vi "deinitialize.vi"(0 "HGF_ImaqFg":refnum<class "HGF_ImaqFg.lvclass">, 5 "error in (no error)":errorcluster) -> (19 "error out":errorcluster)   [LabVIEW 2014, in "HGF_IMAQ.lvlib" / "HGF_ImaqFg.lvclass"]
doc: "This is a dynamic dispatch VI. It can be overwritten by childclasses to release allocated recources."
uses:
  HGF_ImaqFg.lvclass
  HGF_IMAQDevice/HGF_IMAQDevice.lvclass
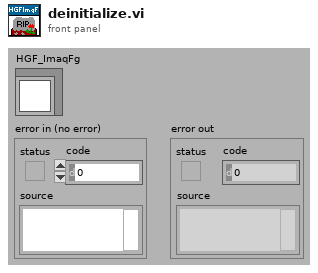
[diagram p1: front panel]
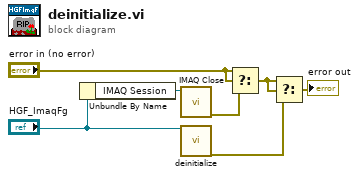
[diagram p0: block diagram]
diagram:
  n1 = Unbundle By Name("HGF_ImaqFg") -> ("IMAQ Session"=w6:refnum<k11>)
  n2 = call <vilib>:"IMAQ Close.vi"("IMAQ Session In"=w6) -> ("error out"=w5:errorcluster)  [unwired: 1 in, 9 out]
  n3 = call-parent "deinitialize.vi"("HGF_IMAQDevice"="HGF_ImaqFg") -> ("error out"=w2:errorcluster)  [unwired: 1 in, 17 out]
  n4 = Select(t="error in (no error)", s="error in (no error)", f=w5) -> (s? t:f=w3:errorcluster)
  n5 = Select(t=w3, s=w3, f=w2) -> (s? t:f=→"error out":errorcluster)
